vi "Init.vi"(10 "Attributes":T1) -> (2 "Attributes":refnum<class "Attributes.lvclass">)   [LabVIEW 2025, in "jettl.lvlib" / "Attributes.lvlib"]
uses:
  Attributes.lvlib
  Attributes/Attributes.lvclass
  Attributes.ctl
  Transport/Transport/Transport.lvclass
  Refs/Refs.lvclass
  Msg Set.ctl
  Msg/Msg.lvclass
  Actor/Actor.lvclass
  Base Attributes/Base Attributes.lvclass
  C:/git/jettl/src/jettl/jettl/Attributes/Attributes/Attributes.lvclass
  jettl.lvlib
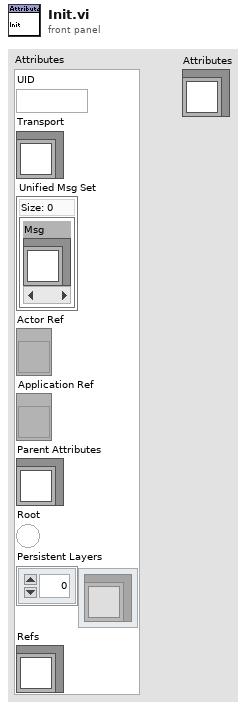
[diagram p1: front panel]
types:
  T1 = typedef "jettl.lvlib/Attributes.ctl" = cluster{"UID":string, "Transport":refnum<class "Transport.lvclass">, "Unified Msg Set":T2, "Actor Ref":refnum<vi>, "Application Ref":refnum<vi>, "Parent Attributes":refnum<class "Attributes.lvclass">, "Root":bool, "Persistent Layers":refnum<class "Actor.lvclass">[], "Refs":refnum<class "Refs.lvclass">}
  T2 = typedef "jettl.lvlib/Msg Set.ctl" = set{refnum<class "Msg.lvclass">}
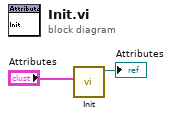
[diagram p0: block diagram]
diagram:
  n1 = call "Init.vi"("Attributes"="Attributes") -> ("Base Attributes out"=→"Attributes":refnum<class "Base Attributes.lvclass">)  [unwired: 10 in]
